vi "Configure3dIndex.vi"(1 "Index Type (Absolute)":T1=1 items=["Incremental", "Absolute", "Registration", "Jog"], 2 "Additional Settings":T2={"Next Index"=0, "Termination"=0, "Count"=1} {"Termination" items=["Stop", "Start Another Immediately", "Start Another x/start Index Input", "Start Another Index Without Stopping"]}, 5 "Index (0)":T5, 7 "Position":T4, 11 "error in (no error)":errorcluster, 12 "Axis Settings":T6=[{"Velocity"=5.0, "Accel. / Decel."=5.0, "Dwell"=0}, {"Velocity"=5.0, "Accel. / Decel."=5.0, "Dwell"=0}, {"Velocity"=5.0, "Accel. / Decel."=5.0, "Dwell"=0}]) -> (6 "Index (duplicate)":T5, 15 "error out":errorcluster)   [LabVIEW 2009]
doc: "Configure an index (motion) on specified axis."
uses:
  typedefs/AxesTestSettings.ctl
  typedefs/Ultra3000/Index_Numeric.ctl
  typedefs/Position3d.ctl
  typedefs/Ultra3000/AdditionalIndexSettings_Cluster.ctl
  typedefs/Ultra3000/IndexTermination.ctl
  typedefs/Ultra3000/IndexType.ctl
  typedefs/Ultra3000/IndexSettings_Cluster.ctl
  typedefs/DwellTime.ctl
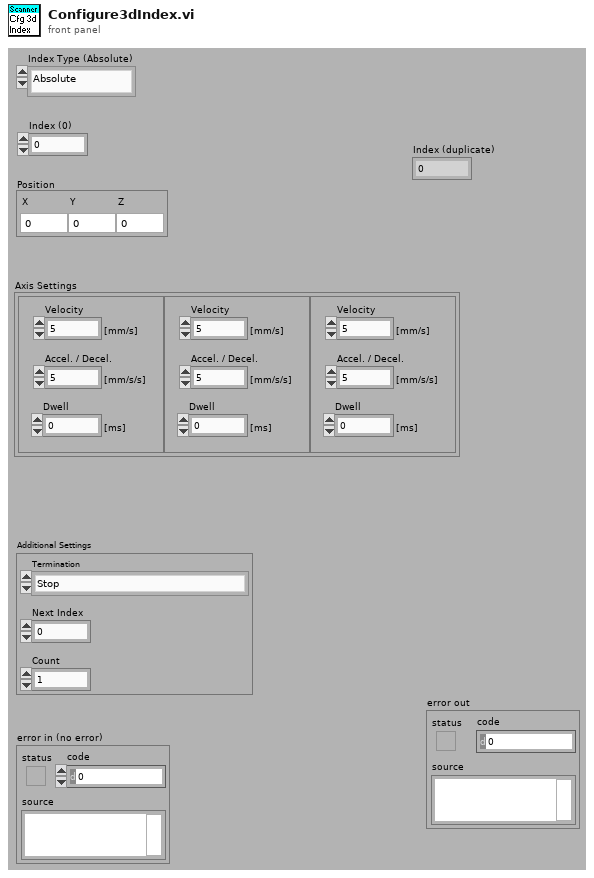
[diagram p1: front panel]
types:
  T1 = typedef "IndexType.ctl" = i32
  T2 = typedef "AdditionalIndexSettings_Cluster.ctl" = cluster{"Next Index":u8, "Termination":T3, "Count":u16}
  T3 = typedef "IndexTermination.ctl" = i32
  T4 = typedef "Position3d.ctl" = cluster{"X":dbl, "Y":dbl, "Z":dbl}
  T5 = typedef "Index_Numeric.ctl" = u8
  T6 = typedef "AxesTestSettings.ctl" = cluster{"Velocity":dbl, "Accel. / Decel.":dbl, "Dwell":u16}[]
  T7 = typedef "IndexSettings_Cluster.ctl" = cluster{"Type":T1, "Dwell":T8, "Velocity":dbl, "Accel/Decel":dbl}
  T8 = typedef "DwellTime.ctl" = u16
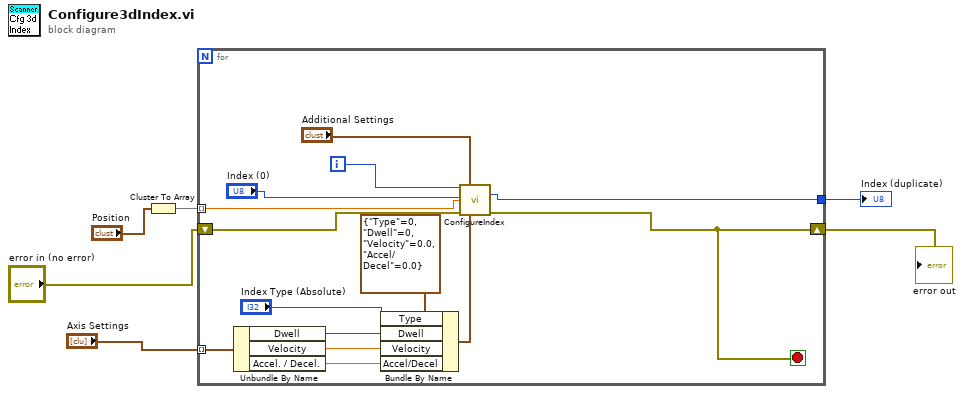
[diagram p0: block diagram]
diagram:
  n1 = Cluster To Array(cluster="Position") -> (array=w4:dbl[])
  n2 = for {
    tunnel: [w20] -> w6
    tunnel: w4 -> [w19] mode=indexing
    tunnel: "Axis Settings" -> [w16] mode=indexing
    shift-right: [w8] -> w1
    shift-left: "error in (no error)" -> [w7]
    i -> [w11]
    stop <- w8 stop-if-true
    n3 = Unbundle By Name(w16) -> ("Dwell"=w15:u16, "Velocity"=w14:dbl, "Accel. / Decel."=w13:dbl)
    n4 = Bundle By Name(cluster=T7 {"Type"=0, "Dwell"=0, "Velocity"=0.0, "Accel/Decel"=0.0} ("Index Settings"), "Type"="Index Type (Absolute)", "Dwell"=w15, "Velocity"=w14, "Accel/Decel"=w13) -> (w18:T7)
    n5 = call "ConfigureIndex.vi"("Axis In"=w11, "Additional Settings"="Additional Settings", "Index (0)"="Index (0)", "Position"=w19, "error in (no error)"=w7, "Index Settings"=w18) -> ("Index (duplicate)"=w20:T5, "error out"=w8:errorcluster)  [unwired: 7 in, 1 out]
  }
  "Index (duplicate)" <- w6
  "error out" <- w1
